vi "IntegrateWaveForm.vi"(4 "First chunk?":bool, 6 "Offset duration":dbl=1.0 format="%0.2f", 7 "Offset correction":dbl, 8 "error in (no error)":errorcluster, 10 "Integrate settings":cluster{"Factor":dbl, "Output name":string}={"Factor"=1.0, "Output name"=""}, 11 "Waveform":waveform(dbl)) -> (0 "error out":errorcluster, 2 "Min max":cluster{"Max":dbl, "Min":dbl}, 3 "Integrated Waveform":waveform(dbl))   [LabVIEW 2015]
uses:
  <vilib>/Analysis/2dsp.llb/Integral Method.ctl
  <vilib>/Analysis/NI_AALPro.lvlib
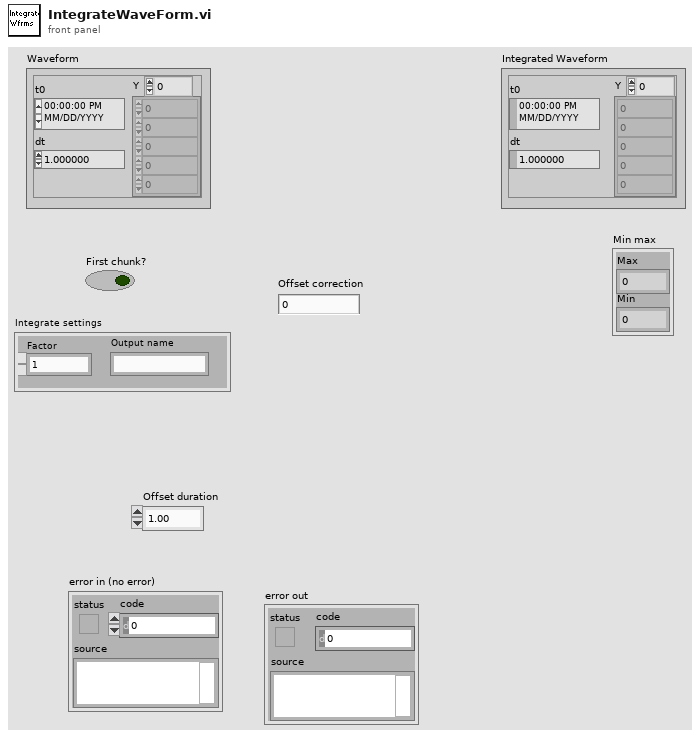
[diagram p1: front panel]
types:
  T1 = typedef "NI_AALPro.lvlib/Integral Method.ctl" = i32
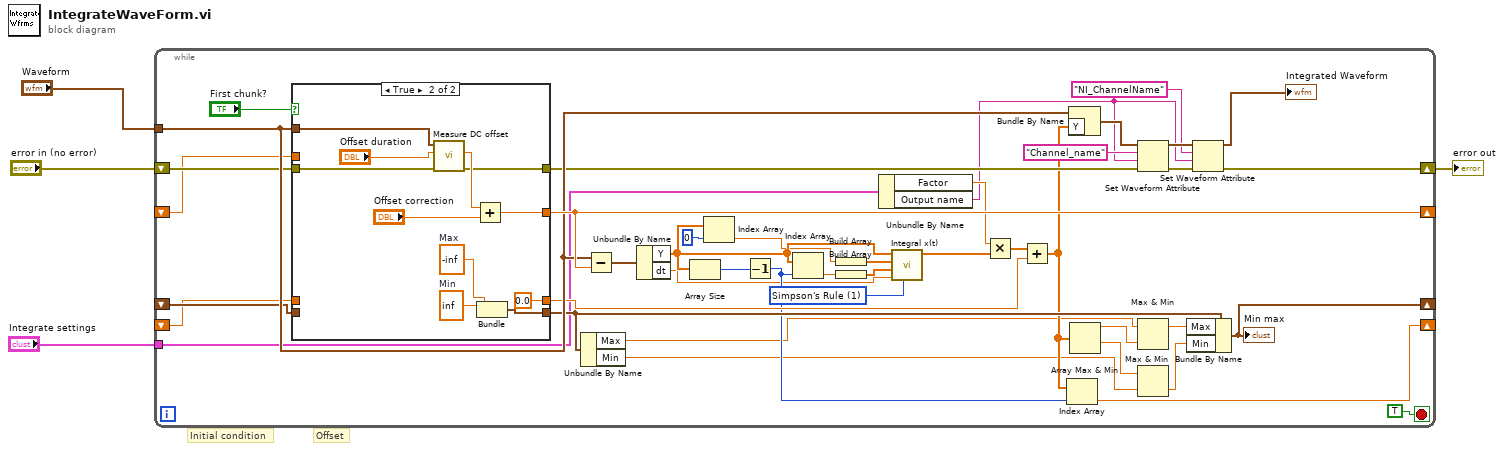
[diagram p0: block diagram]
diagram:
  # "Initial condition"
  # "Offset"
  n1 = while {
    shift-right: [w44] -> _
    shift-left: _ -> [w37]
    shift-right: [w45] -> w3
    shift-left: "error in (no error)" -> [w38]
    shift-right: [w46] -> _
    shift-left: _ -> [w36]
    tunnel: "Waveform" -> [w43]
    shift-right: [w6] -> _
    shift-left: _ -> [w41]
    tunnel: "Integrate settings" -> [w7]
    stop <- TRUE stop-if-true
    w14 = T1 1 items=["Trapezoidal Rule", "Simpson's Rule", "Simpson's 3/8 Rule", "Bode Rule"] ("integration method")
    n2 = case shown="True" "First chunk?" {
      tunnel: [w51 w58] -> w44
      tunnel: w43 -> [_ w52]
      tunnel: w37 -> [w51 _]
      tunnel: w36 -> [w50 _]
      tunnel: [w50 0.0] -> w35
      tunnel: [w48 w53] -> w39
      tunnel: [w49 w61] -> w40
      tunnel: w41 -> [w49 _]
      tunnel: w38 -> [w48 w54]
      frame False {
      }
      frame True {
        w60 = inf  # Min
        w59 = -inf  # Max
        n3 = call "Measure DC offset.vi"("Error In"=w54, "Offset duration"="Offset duration", "Waveform"=w52) -> ("Error Out"=w53:errorcluster, "Offset"=w55:dbl)  [unwired: 7 in]
        n4 = Add(x=w55, y="Offset correction") -> (x+y=w58:dbl)
        n5 = Bundle("Max"=w59, "Min"=w60) -> (w61:cluster{"Max":dbl, "Min":dbl})  [unwired: 1 out]
      }
    }
    n6 = Unbundle By Name(w40) -> ("Max"=w26:dbl, "Min"=w28:dbl)
    n7 = Subtract(x=w43, y=w44) -> (x-y=w34:waveform(dbl))
    n8 = Unbundle By Name(w34) -> ("Y"=w15:dbl[], "dt"=w9:dbl)
    n9 = Array Size(array=w15) -> (size(s)=w32:i32)
    n10 = Index Array(array=w15, index=0) -> (element=w13:dbl)
    n11 = Decrement(x=w32) -> (x-1=w31:i32)
    n12 = Index Array(array=w15, index=w31) -> (element=w11:dbl)
    n13 = Build Array(w13) -> (w12:dbl[])
    n14 = Build Array(w11) -> (w10:dbl[])
    n15 = Unbundle By Name(w7) -> ("Factor"=w17:dbl, "Output name"=w16:string)
    n16 = call <vilib>:"Integral x(t).vi"("integration method"=w14, "dt"=w9, "Final Condition"=w10, "Initial Condition"=w12, "X"=w15) -> ("Integral X"=w8:dbl[])  [unwired: 5 in, 1 out]
    n17 = Multiply(x=w17, y=w8) -> (x*y=w30:dbl[])
    n18 = Add(x=w30, y=w35) -> (x+y=w29:dbl[])
    n19 = Index Array(array=w29, index=w31) -> (element=w46:dbl)
    n20 = Bundle By Name(cluster=w43, "Y"=w29) -> (w22:waveform(dbl))
    n21 = Array Max & Min(array=w29) -> (max value=w25:dbl, min value=w27:dbl)  [unwired: 2 out]
    n22 = Set Waveform Attribute(4:w39, 5:w16, 6:"Channel_name" ("name"), 7:w22) -> (0:w19:errorcluster, 3:w21:waveform(dbl))  [unwired: 1 out]
    n23 = Max & Min(x=w26, y=w25) -> (max(x,y)=w24:dbl)  [unwired: 1 out]
    n24 = Max & Min(x=w27, y=w28) -> (min(x,y)=w23:dbl)  [unwired: 1 out]
    n25 = Bundle By Name(cluster=w40, "Max"=w24, "Min"=w23) -> (w6:cluster{"Max":dbl, "Min":dbl})
    "Min max" <- w6
    n26 = Set Waveform Attribute(4:w19, 5:w16, 6:"NI_ChannelName" ("name"), 7:w21) -> (0:w45:errorcluster, 3:→"Integrated Waveform":waveform(dbl))  [unwired: 1 out]
  }
  "error out" <- w3
